vi "PCM Horizontal Panel.vi"() -> ()   [LabVIEW 2016, in "PCM PanelSplit.lvclass"]
uses:
  PCM PanelSplit.lvclass
  PanelSplitToolkit/PanelObject/PanelObject.lvclass
  <vilib>/Utility/error.llb/DialogType.ctl
  PanelSplitToolkit/PanelDataNode/PanelDataNode.lvclass
  PanelSplitToolkit/PanelDataNode/PanelDataNode.lvclass/PanelDataNode.ctl
  PanelSplitToolkit/QueueManager.llb/CreatQueue.vi
  PanelSplitToolkit/QueueManager.llb/Remove.vi
  PanelSplitToolkit/QueueManager.llb/Insert.vi
  PanelSplitToolkit/QueueManager.llb/Destroy.vi
  PanelSplitToolkit/PanelDataNode/Split Mode.ctl
panel:
  in  "Node*":refnum<data-value>
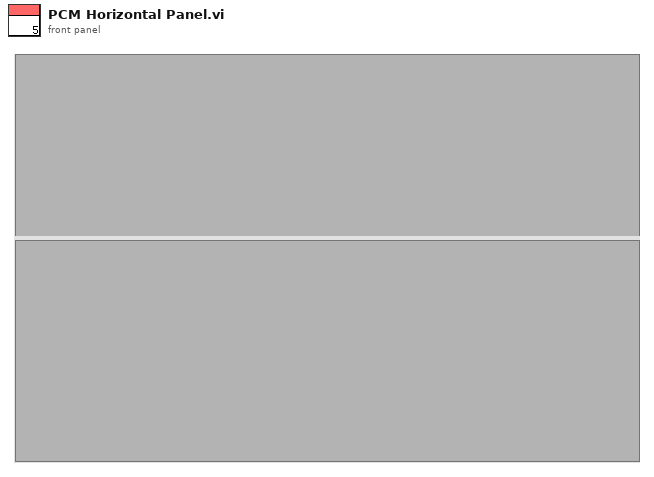
[diagram p1: front panel]
types:
  T1 = cluster{"error":errorcluster, "Event":string, "Data":variant, "Q_Local":string, "Caller":string, "Q_Root":cluster{"Root_QName":string, "Root Event":string, "Root_Data":variant}}
  T2 = typedef "PanelDataNode.lvclass/Split Mode.ctl" = enum16{"Horizontal(up)", "Vertical(left)", "Horizontal(down)", "Vertical(right)"}
  T3 = typedef "DialogType.ctl" = u16
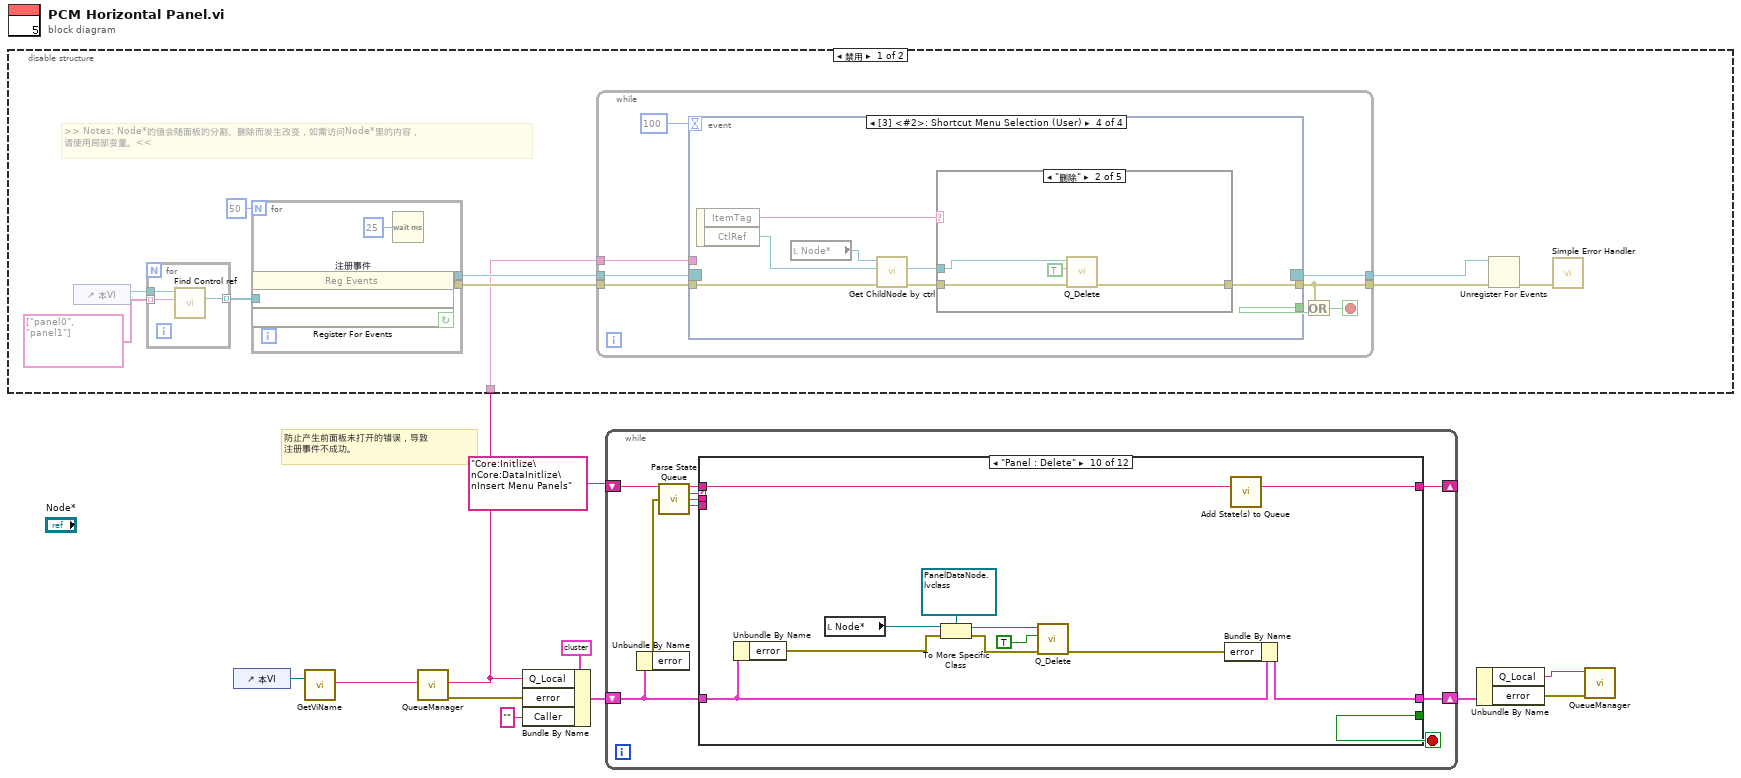
[diagram p0: block diagram]
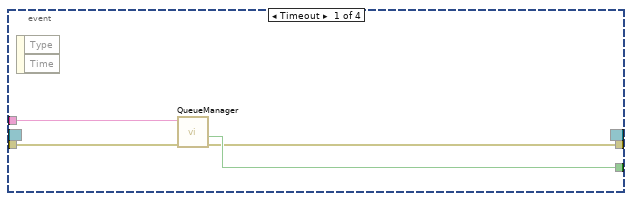
[diagram p2: hidden frame]
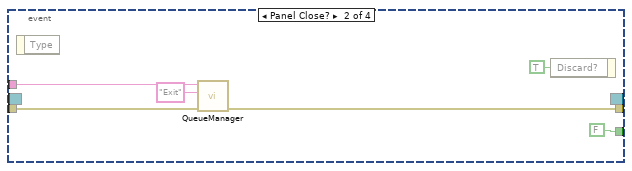
[diagram p3: hidden frame]
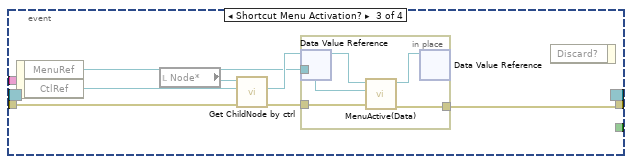
[diagram p4: hidden frame]
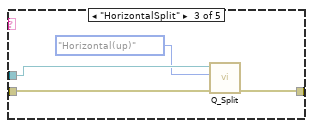
[diagram p6: hidden frame]
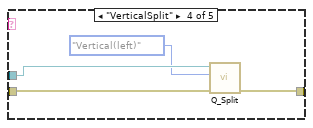
[diagram p7: hidden frame]
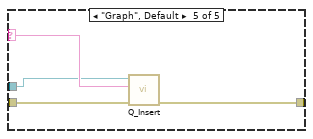
[diagram p8: hidden frame]
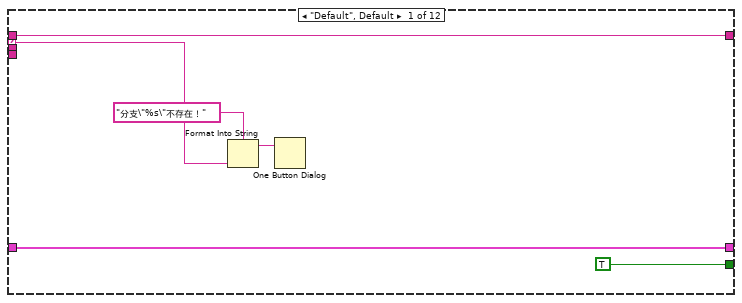
[diagram p10: hidden frame]
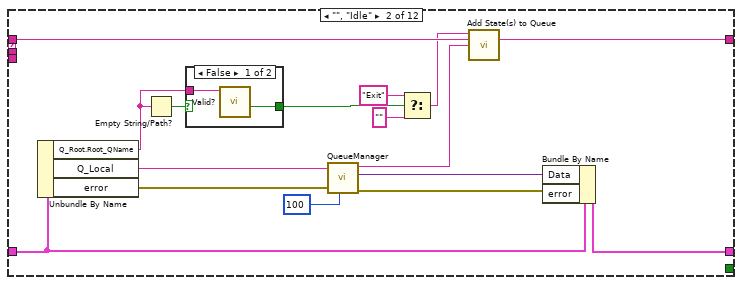
[diagram p11: hidden frame]
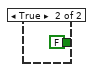
[diagram p12: hidden frame]
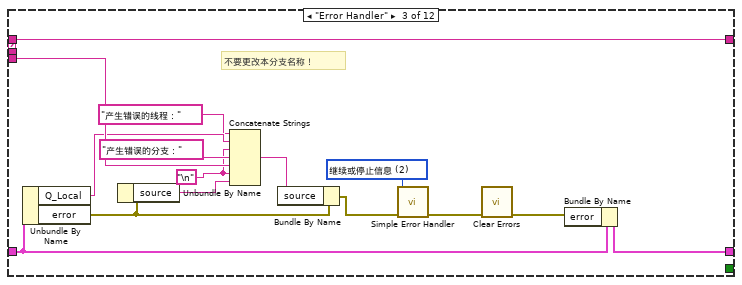
[diagram p13: hidden frame]
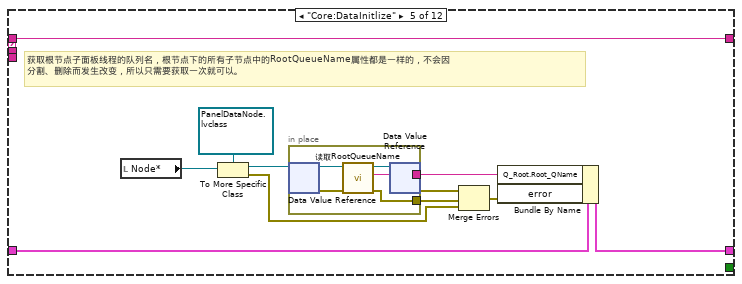
[diagram p15: hidden frame]
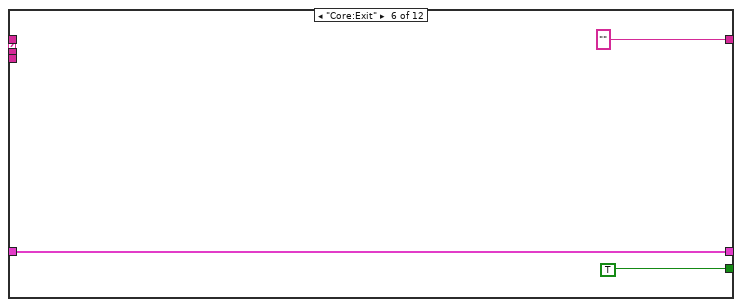
[diagram p16: hidden frame]
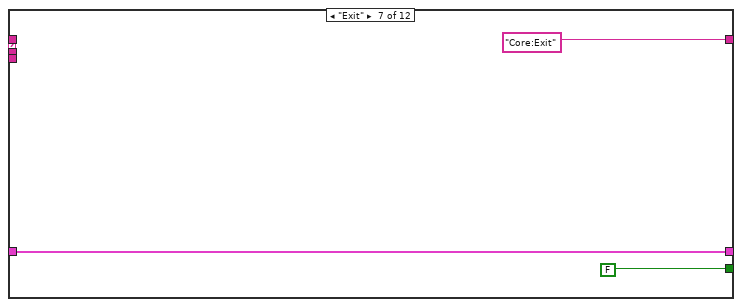
[diagram p17: hidden frame]
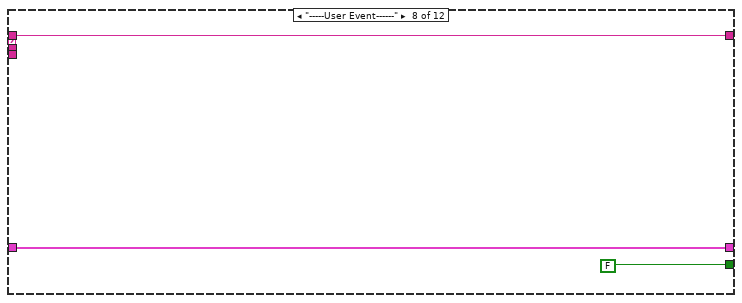
[diagram p18: hidden frame]
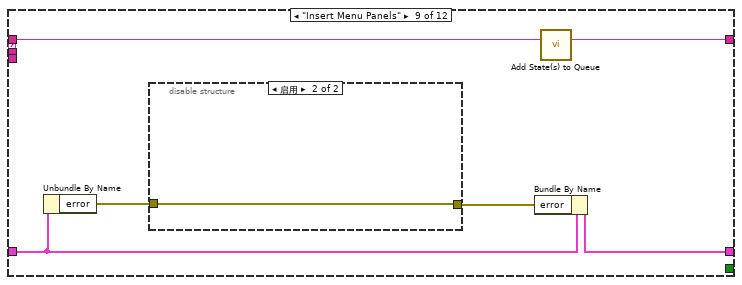
[diagram p19: hidden frame]
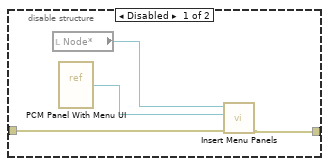
[diagram p20: hidden frame]
diagram:
  # "防止产生前面板未打开的错误，导致\n注册事件不成功。"
  n1 = control-ref of="本VI"() -> (w3:refnum<vi>)
  n2 = call "GetViName.vi"("VI*"=w3) -> ("VI Name"=w1:string)  [unwired: 9 in, 1 out]
  n3 = disable-structure shown="禁用" {
    disable-tunnel: w1 -> [w18 _]
    frame Disabled {
      # ">> Notes: Node*的值会随面板的分割、删除而发生改变，如需访问Node*里的内容，\n请使用局部变量。<<"
      n4 = control-ref of="本VI"() -> (w12:refnum<vi>)
      n5 = for {
        tunnel: w12 -> [w23]
        tunnel: string[] ["panel0", "panel1"] -> [w22] mode=indexing
        tunnel: [w21] -> w17 mode=indexing
        n6 = call "Find Control ref.vi"("control name"=w22, "panelvi*"=w23) -> ("ctrl*"=w21:refnum<vi>)  [unwired: 7 in, 2 out]
      }
      n7 = for {
        N: 50 -> [_]
        tunnel: [w25] -> w20
        tunnel: [w27] -> w19
        tunnel: w17 -> [w26]
        stop <- w25 continue-if-true
        n8 = register-events "注册事件"(w26, w26) -> (reference out=w27:refnum<event-registration>, error out=w25:errorcluster)  [unwired: 2 in]
        n9 = Wait (ms)(milliseconds to wait=u32 25 ("等待时间（毫秒）")) -> ()  [unwired: 1 out]
      }
      n10 = while {
        tunnel: w20 -> [w29]
        tunnel: w18 -> [w35]
        tunnel: [w32] -> w15
        tunnel: w19 -> [w30]
        tunnel: [w28] -> w13
        stop <- w33 stop-if-true
        n11 = event shown="[3] <#2>: Shortcut Menu Selection (User)" {
          selector: w30 -> [_ _ _ _]
          dyn-events: [_ _ _ _] -> w28
          timeout: 100 -> [_ _ _ _]
          tunnel: [w37 FALSE _ _] -> w34
          tunnel: w35 -> [w39 w44 _ _]
          tunnel: w29 -> [w38 w43 w49 w63]
          tunnel: [w36 w42 w47 w61] -> w32
          event Timeout {
            n12 = event-data() -> ()  [unwired: 1 in, 2 out]
            n13 = call-poly "QueueManager.vi"("error in (no error)"=w38, "Queue Name(unamed)"=w39) -> ("error out"=w36:errorcluster, "Not Exist?"=w37:bool)  [unwired: 8 in]
          }
          event Panel Close? {
            n14 = event-data() -> ()  [unwired: 1 in, 1 out]
            n15 = call-poly "QueueManager.vi"("error in"=w43, "Event"="Exit", "QueueName"=w44) -> ("error out"=w42:errorcluster)  [unwired: 7 in, 1 out]
            n16 = event-data("Discard?"=TRUE ("放弃？")) -> ()  [unwired: 1 in, 1 out]
          }
          event Shortcut Menu Activation? {
            n17 = event-data() -> ("MenuRef"=w46:refnum<k9>, "CtlRef"=w50:refnum<vi>)  [unwired: 1 in]
            n18 = local read "Node*"() -> (w51:refnum<data-value>)
            n19 = call "Get ChildNode by ctrl.vi"("error in (no error)"=w49, "ctr*"=w50, "Node*"=w51) -> ("error out"=w48:errorcluster, "ChildNode*"=w52:refnum<data-value>)  [unwired: 7 in]
            n20 = in-place {
              in-place-border: w46 -> [w56]
              in-place-border: w48 -> [w54]
              in-place-border: [w53] -> w47
              n21 = in-place-dvr #1(w52) -> (w57:refnum<class "PanelDataNode.lvclass">)  [unwired: 1 out]
              n22 = call-dynamic "MenuActive(Data).vi"("error in"=w54, "Menu Reference in"=w56, "PanelDataNode in"=w57) -> ("error out"=w53:errorcluster, "PanelDataNode out"=w55:refnum<class "PanelDataNode.lvclass">)  [unwired: 6 in, 1 out]
              n23 = in-place-dvr #1(w55) -> ()  [unwired: 2 out]
            }
            n24 = event-data() -> ()  [unwired: 2 in, 1 out]
          }
          event Shortcut Menu Selection (User) {
            n25 = event-data() -> ("ItemTag"=w60:string, "CtlRef"=w64:refnum<vi>)  [unwired: 1 in]
            n26 = local read "Node*"() -> (w58:refnum<data-value>)
            n27 = call "Get ChildNode by ctrl.vi"("error in (no error)"=w63, "ctr*"=w64, "Node*"=w58) -> ("error out"=w62:errorcluster, "ChildNode*"=w59:refnum<data-value>)  [unwired: 7 in]
            n28 = case shown="\"删除\"" w60 {
              selector: w60 -> [_ _ _ _ w81]
              tunnel: w62 -> [w65 w68 w73 w77 w80]
              tunnel: [w65 w67 w72 w76 w78] -> w61
              tunnel: w59 -> [_ w66 w71 w75 w79]
              frame "假" {
              }
              frame "删除" {
                n29 = call "Q_Delete.vi"("error in"=w68, "CloseVI?(T)"=TRUE, "ChildNode*"=w66) -> ("error out"=w67:errorcluster)  [unwired: 8 in]
              }
              frame "HorizontalSplit" {
                n30 = call "Q_Split.vi"("error in"=w73, "Split Mode"=Split_Mode."Horizontal(up)", "ChildNode*"=w71) -> ("error out"=w72:errorcluster)  [unwired: 8 in]
              }
              frame "VerticalSplit" {
                n31 = call "Q_Split.vi"("error in"=w77, "Split Mode"=Split_Mode."Vertical(left)", "ChildNode*"=w75) -> ("error out"=w76:errorcluster)  [unwired: 8 in]
              }
              frame "Graph", Default {
                n32 = call "Q_Insert.vi"("error in"=w80, "Vi Alias"=w81, "ChildNode*"=w79) -> ("error out"=w78:errorcluster)  [unwired: 8 in]
              }
            }
          }
        }
        n33 = Or(x=w32, y=w34) -> (x .or. y?=w33:bool)
      }
      n34 = Unregister For Events(event registration refnum=w13, error in=w15) -> (error out=w14:errorcluster)
      n35 = call <vilib>:"Simple Error Handler.vi"("error in (no error)"=w14) -> ()  [unwired: 4 in, 5 out]
    }
    frame Enabled {
    }
  }
  n36 = call-poly "QueueManager.vi"("QueueName"=w1) -> ("error out"=w2:errorcluster)  [unwired: 9 in, 1 out]
  n37 = Bundle By Name(cluster=T1 {"error"={"status"=FALSE, "code"=0, "source"=""}, "Event"="", "Data"=variant, "Q_Local"="", "Caller"="", "Q_Root"={"Root_QName"="", "Root Event"="", "Root_Data"=variant}} ("TmpData"), "Q_Local"=w1, "error"=w2, "Caller"="") -> (w6:T1)
  n38 = while {
    shift-right: [w85] -> w8
    shift-left: w6 -> [w86]
    shift-right: [w84] -> _
    shift-left: "Core:Initlize\nCore:DataInitlize\nInsert Menu Panels" -> [w91]
    stop <- w88 stop-if-true
    n39 = Unbundle By Name(w86) -> ("error"=w87:errorcluster)
    n40 = call "Parse State Queue.vi"("State Queue"=w91, "Error In (no error)"=w87) -> ("Remaining States"=w90:string, "Current State"=w89:string, "Arguments"=w83:string, "PreState"=w82:string)  [unwired: 10 in]
    n41 = case shown="\"Panel : Delete\"" w89 {
      selector: w89 -> [w95 _ _ _ _ _ _ _ _ _ _ _]
      tunnel: w90 -> [w96 w110 w131 w133 w144 _ _ w156 w162 w178 w181 w190]
      tunnel: w83 -> [_ _ _ _ _ _ _ _ _ _ _ _]
      tunnel: [TRUE _ _ _ _ TRUE FALSE FALSE _ _ _ _] -> w88
      tunnel: w86 -> [w97 w107 w128 w132 w140 w151 w154 w157 w163 w179 w182 w184]
      tunnel: [w97 w112 w127 w132 w139 w151 w154 w157 w164 w180 w182 w183] -> w85
      tunnel: [w96 w109 w131 w133 w144 "" ("Remaining States") "Core:Exit" ("Remaining States") w156 w161 w177 w181 w190] -> w84
      tunnel: w82 -> [_ _ w125 _ _ _ _ _ _ _ _ _]
      frame "Default", Default {
        n42 = Format Into String(format string="分支\"%s\"不存在！" ("格式字符串"), w95) -> (resulting string=w94:string)  [unwired: 2 in, 1 out]
        n43 = One Button Dialog(message=w94) -> ()  [unwired: 1 in, 1 out]
      }
      frame "", "Idle" {
        n44 = Unbundle By Name(w107) -> ("Q_Root.Root_QName"=w101:string, "Q_Local"=w106:string, "error"=w105:errorcluster)
        n45 = Empty String/Path?(string/path=w101) -> (empty?=w104:bool)
        n46 = case shown="False" w104 {
          tunnel: [w115 FALSE ("Not Exist?")] -> w103
          tunnel: w101 -> [w114 _]
          frame False {
            n47 = call "Valid?.vi"("Queue Name(unamed)"=w114) -> ("Not Exist?"=w115:bool)  [unwired: 9 in, 1 out]
          }
          frame True {
          }
        }
        n48 = call-poly "QueueManager.vi"("Time out(-1)"=100, "error in (no error)"=w105, "Queue Name"=w106) -> ("error out"=w113:errorcluster, "Data"=w111:variant, "Event"=w100:string)  [unwired: 5 in, 1 out]
        n49 = Select(t="Exit" ("Event"), s=w103, f="") -> (s? t:f=w98:string)
        n50 = call "Add State(s) to Queue.vi"("State(s) in Front (\"\")"=w98, "State(s) in (\"\")"=w110, "State(s) at Back (\"\")"=w100) -> ("States Out"=w109:string)  [unwired: 12 in]
        n51 = Bundle By Name(cluster=w107, "Data"=w111, "error"=w113) -> (w112:T1)
      }
      frame "Error Handler" {
        w118 = "\n"
        w126 = T3 2 items=["无对话框", "确定信息", "继续或停止信息", "确定信息＋警告", "继续/停止+警告"] ("type of dialog (OK msg:1)")
        # "不要更改本分支名称！"
        n52 = Unbundle By Name(w128) -> ("Q_Local"=w119:string, "error"=w121:errorcluster)
        n53 = Unbundle By Name(w121) -> ("source"=w123:string)
        n54 = Concatenate Strings("产生错误的线程：" ("字符串"), w119, w118, "产生错误的分支：" ("字符串"), w125, w118, w123) -> (w122:string)
        n55 = Bundle By Name(cluster=w121, "source"=w122) -> (w120:errorcluster)
        n56 = call <vilib>:"Simple Error Handler.vi"("type of dialog (OK msg:1)"=w126, "error in (no error)"=w120) -> ("error out"=w129:errorcluster)  [unwired: 3 in, 4 out]
        n57 = call <vilib>:"Clear Errors.vi"("error in (no error)"=w129) -> ("error out"=w130:errorcluster)  [unwired: 5 in, 1 out]
        n58 = Bundle By Name(cluster=w128, "error"=w130) -> (w127:T1)
      }
      frame "Core:Initlize" {
      }
      frame "Core:DataInitlize" {
        # "获取根节点子面板线程的队列名，根节点下的所有子节点中的RootQueueName属性都是一样的，不会因\n分割、删除而发生改变，所以只需要获取一次就可以。"
        n59 = local read "Node*"() -> (w141:refnum<data-value>)
        n60 = To More Specific Class(target class=refnum<data-value> refnum ("Node*"), reference=w141) -> (specific class reference=w143:refnum<data-value>, error out=w134:errorcluster)  [unwired: 1 in]
        n61 = in-place {
          in-place-border: [w146] -> w138
          in-place-border: [w145] -> w137
          n62 = in-place-dvr #2(w143) -> (w149:refnum<class "PanelDataNode.lvclass">, w147:errorcluster)
          n63 = call "读取RootQueueName.vi"("error in (no error)"=w147, "PanelDataNode输入"=w149) -> ("error out"=w145:errorcluster, "RootQueueName"=w146:string, "PanelDataNode输出"=w148:refnum<class "PanelDataNode.lvclass">)  [unwired: 7 in]
          n64 = in-place-dvr #2(w148) -> (w136:errorcluster)  [unwired: 1 out]
        }
        n65 = Merge Errors(w136, w137, w134) -> (w135:errorcluster)
        n66 = Bundle By Name(cluster=w140, "Q_Root.Root_QName"=w138, "error"=w135) -> (w139:T1)
      }
      frame "Core:Exit" {
      }
      frame "Exit" {
      }
      frame "-----User Event------" {
      }
      frame "Insert Menu Panels" {
        n67 = Unbundle By Name(w163) -> ("error"=w159:errorcluster)
        n68 = disable-structure shown="启用" {
          disable-tunnel: [w168 w169] -> w160
          disable-tunnel: w159 -> [w167 w169]
          frame Disabled {
            n69 = local read "Node*"() -> (w165:refnum<data-value>)
            n70 = vi-ref "PCM Panel With Menu UI.vi"() -> (w166:refnum<vi>)
            n71 = call "Insert Menu Panels.vi"("错误输入"=w167, "Static VI*"=w166, "Node*"=w165) -> ("error out"=w168:errorcluster)  [unwired: 8 in]
          }
          frame Enabled {
          }
        }
        n72 = Bundle By Name(cluster=w163, "error"=w160) -> (w164:T1)
        n73 = call "Add State(s) to Queue.vi"("State(s) in (\"\")"=w162) -> ("States Out"=w161:string)  [unwired: 14 in]
      }
      frame "Panel : Delete" {
        n74 = Unbundle By Name(w179) -> ("error"=w172:errorcluster)
        n75 = local read "Node*"() -> (w170:refnum<data-value>)
        n76 = To More Specific Class(target class=refnum<data-value> refnum ("Node*"), reference=w170, error in=w172) -> (specific class reference=w175:refnum<data-value>, error out=w173:errorcluster)
        n77 = call "Q_Delete.vi"("error in"=w173, "CloseVI?(T)"=TRUE, "ChildNode*"=w175) -> ("error out"=w171:errorcluster)  [unwired: 8 in]
        n78 = Bundle By Name(cluster=w179, "error"=w171) -> (w180:T1)
        n79 = call "Add State(s) to Queue.vi"("State(s) in (\"\")"=w178) -> ("States Out"=w177:string)  [unwired: 14 in]
      }
      frame "---Communication----" {
      }
      frame "Com : Send To RootQ" {
        n80 = Unbundle By Name(w184) -> ("Q_Root.Root_QName"=w186:string, "Q_Root.Root Event"=w187:string, "Q_Root.Root_Data"=w188:variant, "error"=w189:errorcluster)
        n81 = call-poly "QueueManager.vi"("error in"=w189, "Data"=w188, "Event"=w187, "QueueName"=w186) -> ("error out"=w185:errorcluster)  [unwired: 6 in, 1 out]
        n82 = Bundle By Name(cluster=w184, "error"=w185) -> (w183:T1)
      }
    }
  }
  n83 = Unbundle By Name(w8) -> ("Q_Local"=w5:string, "error"=w9:errorcluster)
  n84 = call-poly "QueueManager.vi"("error in (no error)"=w9, "QueeuName"=w5) -> ()  [unwired: 9 in, 1 out]
